vi "Result.Numeric Limits to String Items for Results Table.vi"(6 "N/A Filler":string="n/a", 8 "UL":dbl, 9 "LL":dbl, 10 "LimType":T1, 11 "Value":dbl) -> (0 "UL":string, 1 "LL":string, 2 "LimType":string, 3 "Value":string)   [LabVIEW 2018]
uses:
  Result.Limit Type.ctl
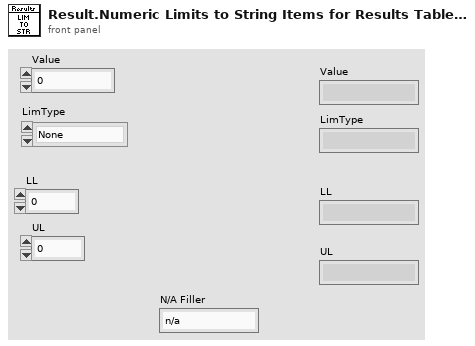
[diagram p1: front panel]
types:
  T1 = typedef "Result.Limit Type.ctl" = enum16{"None", "EQ", "NE", "GT", "LT", "GE", "LE", "GTLT", "GELE", "GELT", "GTLE", "LTGT", "LEGE", "LEGT", "LTGE", "Contains", "NotContains"}
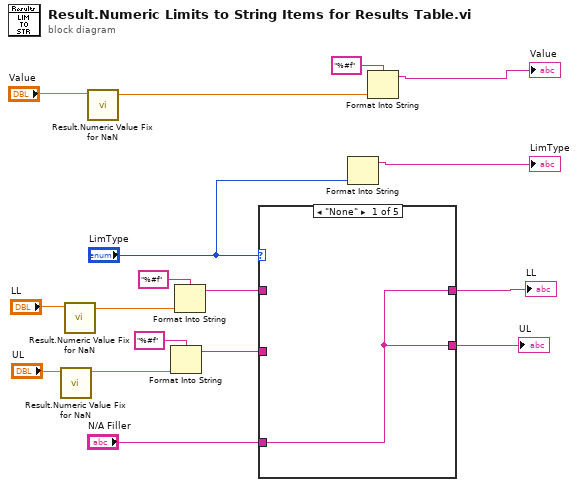
[diagram p0: block diagram]
diagram:
  n1 = call "Result.Numeric Value Fix for NaN.vi"("Numeric"="UL") -> ("Numeric Out"=w3:dbl)  [unwired: 10 in]
  n2 = call "Result.Numeric Value Fix for NaN.vi"("Numeric"="LL") -> ("Numeric Out"=w2:dbl)  [unwired: 10 in]
  n3 = call "Result.Numeric Value Fix for NaN.vi"("Numeric"="Value") -> ("Numeric Out"=w1:dbl)  [unwired: 10 in]
  n4 = Format Into String(format string="%#f", w3) -> (resulting string=w14:string)  [unwired: 2 in, 1 out]
  n5 = Format Into String(format string="%#f", w2) -> (resulting string=w15:string)  [unwired: 2 in, 1 out]
  n6 = case shown="\"None\"" "LimType" {
    tunnel: w15 -> [_ w20 w22 _ w25]
    tunnel: w14 -> [_ _ _ w23 w26]
    tunnel: "N/A Filler" -> [w18 w19 w21 w24 _]
    tunnel: [w18 w20 w22 w24 w25] -> w10
    tunnel: [w18 w19 w21 w23 w26] -> w9
    frame "None" {
    }
    frame "EQ".."GT", "GE" {
    }
    frame "Contains", "NotContains" {
    }
    frame "LT", "LE" {
    }
    frame Default {
    }
  }
  "LL" <- w10
  "UL" <- w9
  n7 = Format Into String("LimType") -> (resulting string=→"LimType":string)  [unwired: 3 in, 1 out]
  n8 = Format Into String(format string="%#f", w1) -> (resulting string=→"Value":string)  [unwired: 2 in, 1 out]
